vi "Get_Firmware.vi"(8 "error in":errorcluster, 11 "VISA name":refnum<visa-resource-name>) -> (0 "error out":errorcluster, 1 "valid":bool, 2 "FW":string, 3 "VISA out":refnum<visa-resource-name>)   [LabVIEW 2023, in "QR 10X Eastwood.lvlib"]
uses:
  <instrlib>/QR 10X Eastwood/QR 10X Eastwood.lvlib
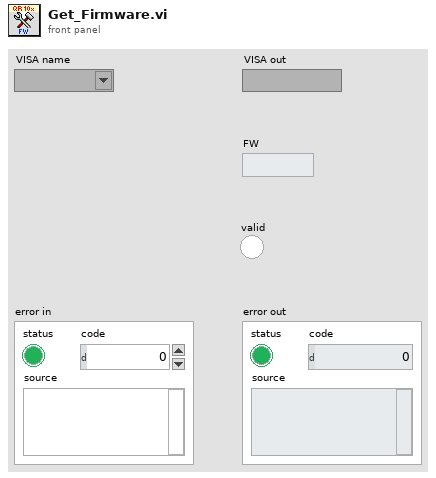
[diagram p1: front panel]
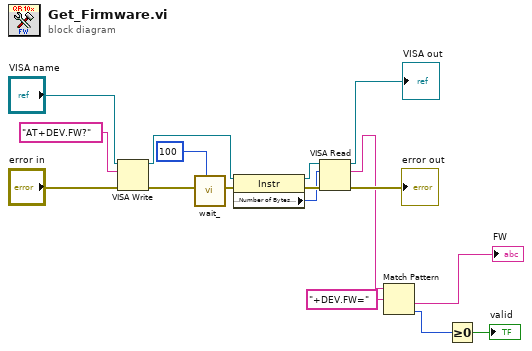
[diagram p0: block diagram]
diagram:
  n1 = VISA Write(VISA resource name="VISA name", write buffer="AT+DEV.FW?", error in (no error)="error in") -> (VISA resource name out=w13:refnum<visa-resource-name>, error out=w8:errorcluster)  [unwired: 1 out]
  n2 = call "wait_.vi"("milliseconds to wait"=u32 100, "error in"=w8) -> ("error out"=w7:errorcluster)  [unwired: 9 in]
  n3 = property class="Instr"(reference=w13, error in=w7) -> (reference out=w9:refnum<visa-resource-name>, error out=w11:errorcluster, "Serial Settings:Number of Bytes at Serial Port"=w10:u32)
  n4 = VISA Read(VISA resource name=w9, byte count=w10, error in (no error)=w11) -> (VISA resource name out=→"VISA out":refnum<visa-resource-name>, read buffer=w5:string, error out=→"error out":errorcluster)  [unwired: 1 out]
  n5 = Match Pattern(string=w5, regular expression="+DEV.FW=") -> (after substring=→"FW":string, offset past match=w2:i32)  [unwired: 1 in, 2 out]
  n6 = Greater Or Equal To 0?(x=w2) -> (x >= 0?=→"valid":bool)
